vi "A4988_for_stm32.vi"() -> ()   [LabVIEW 2015]
uses:
  <vilib>/Instr/_visa.llb/VISA Configure Serial Port (Instr).vi
panel:
  in  "VISA resource name":refnum<visa-resource-name>
  out "String":string
  in  "Boolean":bool
  in  "stop":bool
  out "Current position":dbl
  in  "?":u64(knob)=1 min=1 max=16 scale=1.0..16.0
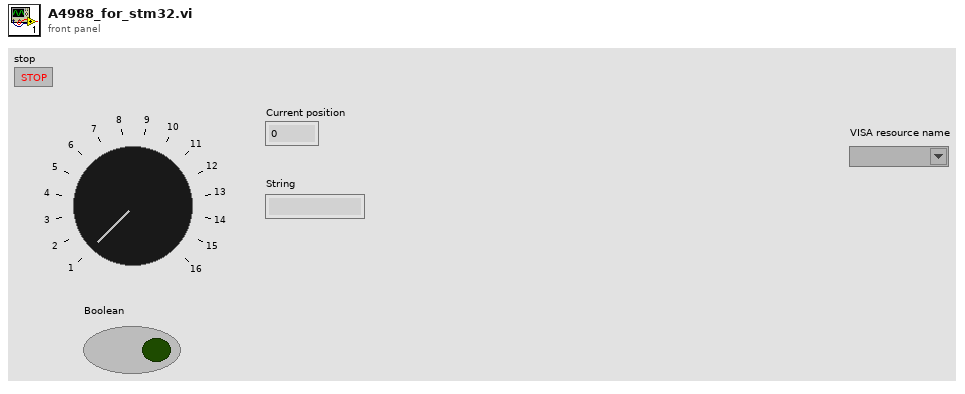
[diagram p1: front panel]
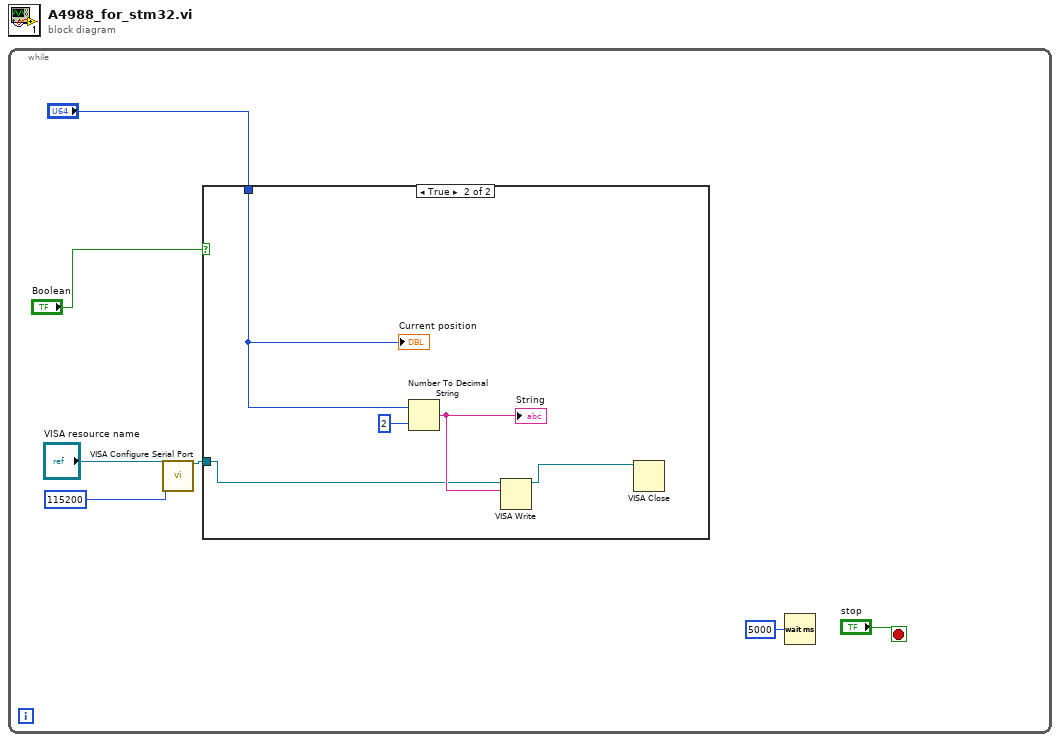
[diagram p0: block diagram]
diagram:
  n1 = while {
    stop <- "stop" stop-if-true
    n2 = call-poly "VISA Configure Serial Port"("VISA resource name"="VISA resource name", "baud rate (9600)"=u32 115200) -> ("VISA resource name out"=w3:refnum<visa-resource-name>)  [unwired: 12 in, 1 out]
    n3 = case shown="True" "Boolean" {
      tunnel: "?" -> [_ w11]
      tunnel: w3 -> [_ w8]
      frame False {
      }
      frame True {
        n4 = Number To Decimal String(number=w11, width (-)=i16 2) -> (decimal integer string=w10:string)
        "String" <- w10
        n5 = VISA Write(VISA resource name=w8, write buffer=w10) -> (VISA resource name out=w9:refnum<visa-resource-name>)  [unwired: 1 in, 2 out]
        n6 = VISA Close(VISA resource name=w9) -> ()  [unwired: 1 in, 1 out]
        "Current position" <- w11
      }
    }
    n7 = Wait (ms)(milliseconds to wait=u32 5000) -> ()  [unwired: 1 out]
  }
